vi "Translate sphere.vi"(1 "Translation vector (dx, dy, dz)":sgl[](array[numeric]), 2 "Sphere in":T1) -> (0 "Sphere out":T1)   [LabVIEW 2014]
uses:
  Typedefs/Sphere.ctl
panel:
  # "PN 13/03/2015"
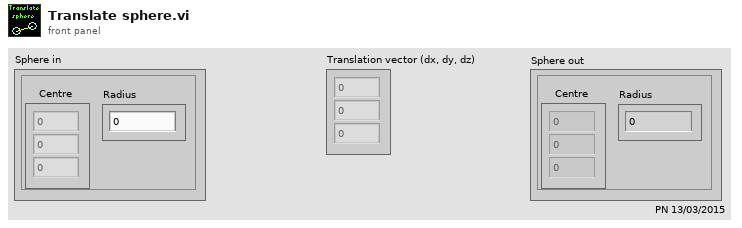
[diagram p1: front panel]
types:
  T1 = typedef "Sphere.ctl" = cluster{"Centre":sgl[], "Radius":sgl}
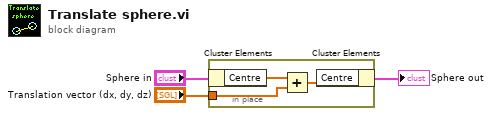
[diagram p0: block diagram]
diagram:
  n1 = in-place {
    in-place-border: "Translation vector (dx, dy, dz)" -> [w4]
    n2 = in-place-cluster #1("Sphere in") -> ("Centre"=w6:sgl[])
    n3 = Add(x=w6, y=w4) -> (x+y=w5:sgl[])
    n4 = in-place-cluster #1("Centre"=w5) -> (→"Sphere out":T1)
  }
